vi "executeQuery.vi"(8 "error in (no error)":errorcluster, 10 "command":string, 11 "Electrometer in":refnum<class "Electrometer.lvclass">) -> (0 "error out":errorcluster, 2 "result":string, 3 "Electrometer out":refnum<class "Electrometer.lvclass">)   [LabVIEW 2016, in "Electrometer.lvclass"]
uses:
  Electrometer.lvclass
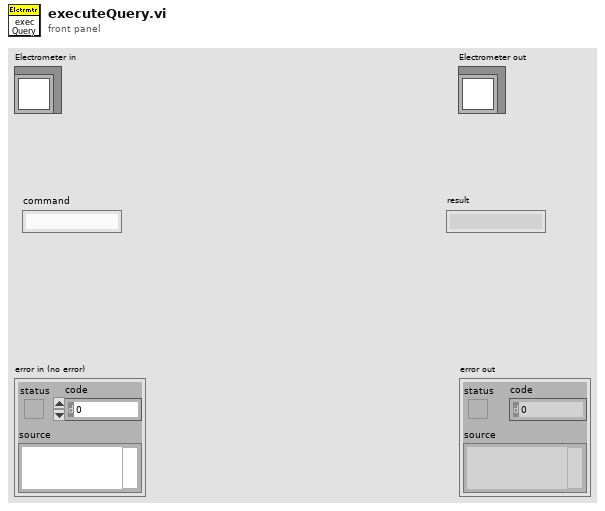
[diagram p1: front panel]
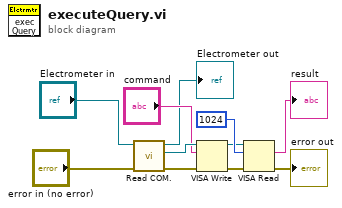
[diagram p0: block diagram]
diagram:
  n1 = call "Read COM..vi"("error in (no error)"="error in (no error)", "Electrometer in"="Electrometer in") -> ("error out"=w11:errorcluster, "VISA"=w10:refnum<visa-resource-name>, "Electrometer out"=→"Electrometer out":refnum<class "Electrometer.lvclass">)  [unwired: 7 in]
  n2 = VISA Write(VISA resource name=w10, write buffer="command", error in (no error)=w11) -> (VISA resource name out=w3:refnum<visa-resource-name>, error out=w4:errorcluster)  [unwired: 1 out]
  n3 = VISA Read(VISA resource name=w3, byte count=u32 1024, error in (no error)=w4) -> (read buffer=→"result":string, error out=→"error out":errorcluster)  [unwired: 2 out]
